vi "Read.vi"(9 "timeout in ms (-1)":i32=-1, 11 "Lossless in":refnum<class "Lossless.lvclass">) -> (0 "error out":errorcluster, 1 "timed out?":bool, 2 "Element":T1, 3 "Lossless out":refnum<class "Lossless.lvclass">)   [LabVIEW 2022 SP3, in "Enclave.lvlib" / "Lossless.lvclass"]
uses:
  Lossless.lvclass
  Element.ctl
  Lossless.lvclass/Lossless.ctl
  Enclave.lvlib
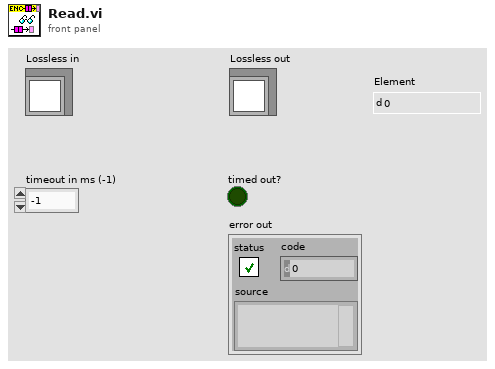
[diagram p1: front panel]
types:
  T1 = typedef "Enclave.lvlib/Element.ctl" = dbl
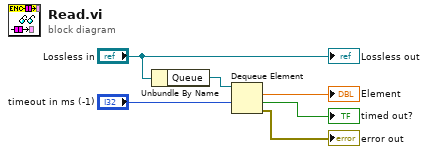
[diagram p0: block diagram]
diagram:
  n1 = Unbundle By Name("Lossless in") -> ("Queue"=w5:refnum<queue>)
  n2 = Dequeue Element(queue=w5, timeout in ms (-1)="timeout in ms (-1)") -> (element=→"Element":T1, timed out?=→"timed out?":bool, error out=→"error out":errorcluster)  [unwired: 1 in, 1 out]
  "Lossless out" <- "Lossless in"
